vi "ConfigureSweepCoupling.vi"(8 "error in (no error)":errorcluster, 11 "SpecAnBase in":refnum<class "SpecAnBase.lvclass">) -> (0 "error out":errorcluster, 3 "SpecAnBase out":refnum<class "SpecAnBase.lvclass">)   [LabVIEW 2014, in "SpecAnPlugins.lvlib" / "SpecAnBase.lvclass"]
doc: "This function configures the coupling and sweeping attributes such as sweep time (time it takes to go from the start frequency to the stop frequency), Resolution Bandwidthm, and the Video Bandwidth."
uses:
  SpecAnBase.lvclass
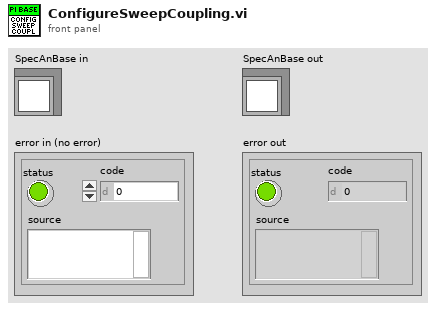
[diagram p1: front panel]
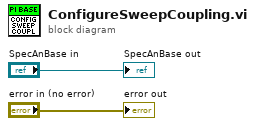
[diagram p0: block diagram]
diagram:
  "error out" <- "error in (no error)"
  "SpecAnBase out" <- "SpecAnBase in"
